vi "Get Picture.vi"(8 "error in (no error)":errorcluster, 11 "Small Register Bank in":refnum<class "Small Register Bank.lvclass">) -> (0 "error out":errorcluster, 2 "Picture":picture, 3 "Small Register Bank out":refnum<class "Small Register Bank.lvclass">)   [LabVIEW 2020, in "Small Register Bank.lvclass"]
uses:
  Small Register Bank.lvclass
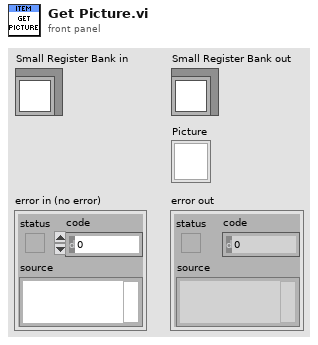
[diagram p1: front panel]
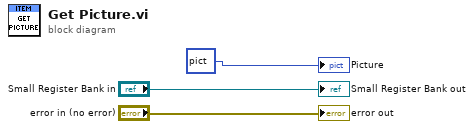
[diagram p0: block diagram]
diagram:
  "error out" <- "error in (no error)"
  "Small Register Bank out" <- "Small Register Bank in"
  "Picture" <- picture bytes[3230] ("new picture")
